vi "Over Threshold.vi"(8 "error in (no error)":errorcluster, 11 "UI in":refnum<class "UI.lvclass">) -> (0 "error out":errorcluster, 3 "UI out":refnum<class "UI.lvclass">)   [LabVIEW 2020, in "UI.lvlib" / "UI.lvclass"]
uses:
  UI.lvclass
  UI.lvclass/UI.ctl
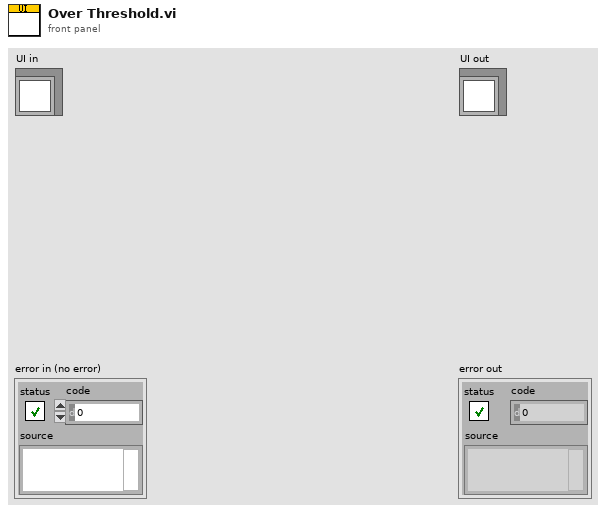
[diagram p1: front panel]
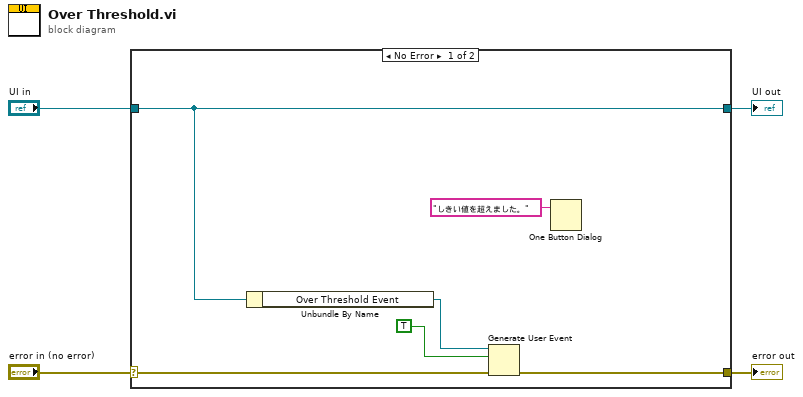
[diagram p0: block diagram]
diagram:
  n1 = case shown="No Error" "error in (no error)" {
    selector: "error in (no error)" -> [w6 w12]
    tunnel: [w5 w12] -> w3
    tunnel: [w9 w11] -> w1
    tunnel: "UI in" -> [w9 w11]
    frame No Error {
      n2 = Unbundle By Name(w9) -> ("Over Threshold Event"=w8:refnum<user-event>)
      n3 = Generate User Event(user event=w8, event data cluster=TRUE ("event data"), error in=w6) -> (error out=w5:errorcluster)  [unwired: 1 in, 1 out]
      n4 = One Button Dialog(message="しきい値を超えました。") -> ()  [unwired: 1 in, 1 out]
    }
    frame Error {
    }
  }
  "error out" <- w3
  "UI out" <- w1
